vi "SM Destroy Event.vi"(8 "error in (no error)":errorcluster, 11 "Req. Transition Event":refnum<user-event>) -> (0 "error out":errorcluster)   [LabVIEW 2022 SP3, in "StateMachine.lvlib" / "HSE-State-Machine.lvlib"]
doc: "Destroys the local user event used for requesting a transition.\n\n____\nHAMPEL SOFTWARE ENGINEERING v2.6.0 (2023-12-19 10:54)"
uses:
  HSE-State-Machine.lvlib
  SM Request Transition Argument--cluster.ctl
  SM_Transitions.ctl
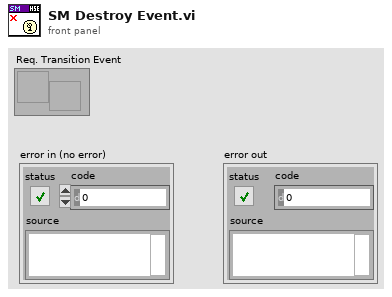
[diagram p1: front panel]
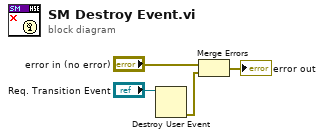
[diagram p0: block diagram]
diagram:
  n1 = Destroy User Event(user event="Req. Transition Event") -> (error out=w2:errorcluster)  [unwired: 1 in]
  n2 = Merge Errors("error in (no error)", w2) -> (→"error out":errorcluster)
